vi "DAQmx.Stop.vi"(8 "error in (no error)":errorcluster, 11 "DAQmx in":refnum<class "DAQmx.lvclass">) -> (0 "error out":errorcluster, 3 "DAQmx out":refnum<class "DAQmx.lvclass">)   [LabVIEW 2019, in "DAQmx.lvclass"]
uses:
  DAQmx.lvclass
  DAQmx.lvclass/DAQmx.ctl
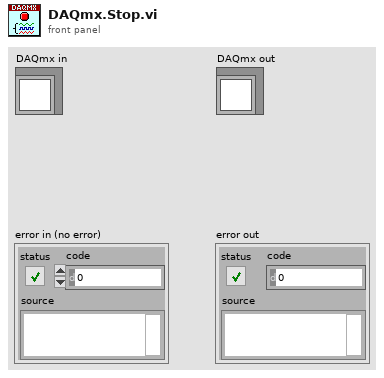
[diagram p1: front panel]
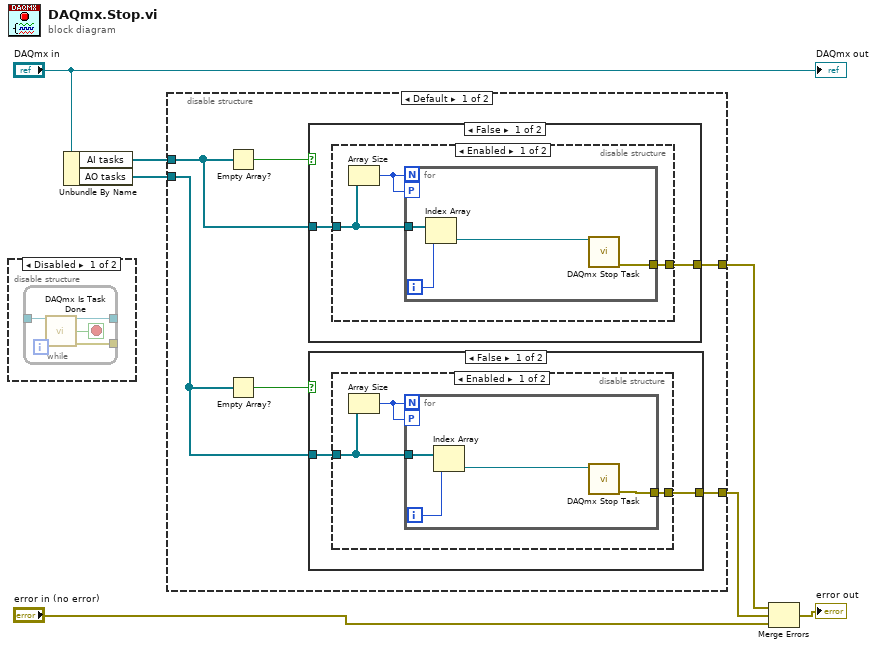
[diagram p0: block diagram]
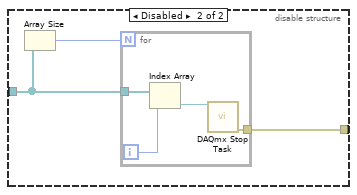
[diagram p3: hidden frame]
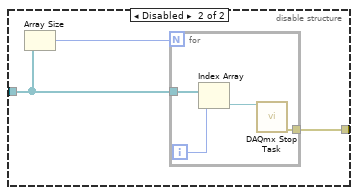
[diagram p5: hidden frame]
diagram:
  n1 = disable-structure shown="Disabled" {
    frame Disabled {
      n2 = while {
        tunnel: [w9] -> _
        tunnel: _ -> [w11]
        tunnel: [w10] -> _
        stop <- w8 stop-if-true
        n3 = call <vilib>:"DAQmx Is Task Done.vi"("task/channels in"=w11) -> ("task out"=w10:refnum<k21>, "task done?"=w8:bool, "error out"=w9:errorcluster)  [unwired: 12 in]
      }
    }
    frame Enabled {
    }
  }
  n4 = Unbundle By Name("DAQmx in") -> ("AI tasks"=w6:refnum<k21>[], "AO tasks"=w7:refnum<k21>[])
  n5 = disable-structure shown="Default" {
    disable-tunnel: [w17 _] -> w3
    disable-tunnel: w7 -> [w13 _]
    disable-tunnel: w6 -> [w15 _]
    disable-tunnel: [w12 _] -> w1
    frame condition #0 (active) {
      n6 = Empty Array?(array=w15) -> (empty?=w16:bool)
      n7 = Empty Array?(array=w13) -> (empty?=w14:bool)
      n8 = case shown="False" w16 {
        tunnel: w15 -> [w34 _]
        tunnel: [w35 _] -> w17
        frame False {
          n9 = disable-structure shown="Enabled" {
            disable-tunnel: [w38 w45] -> w35
            disable-tunnel: w34 -> [w37 w44]
            frame Enabled {
              n10 = Array Size(array=w37) -> (size(s)=w36:i32)
              n11 = for {
                N: w36 -> [_]
                tunnel: w37 -> [w41]
                tunnel: [w42] -> w38
                workers-P: w36 -> [_]
                i -> [w40]
                n12 = Index Array(array=w41, index=w40) -> (element=w39:refnum<k21>)
                n13 = call <vilib>:"DAQmx Stop Task.vi"("task/channels in"=w39) -> ("error out"=w42:errorcluster)  [unwired: 13 in, 1 out]
              }
            }
            frame Disabled {
              n14 = Array Size(array=w44) -> (size(s)=w43:i32)
              n15 = for {
                N: w43 -> [_]
                tunnel: w44 -> [w48]
                tunnel: [w49] -> w45
                i -> [w47]
                n16 = Index Array(array=w48, index=w47) -> (element=w46:refnum<k21>)
                n17 = call <vilib>:"DAQmx Stop Task.vi"("task/channels in"=w46) -> ("error out"=w49:errorcluster)  [unwired: 13 in, 1 out]
              }
            }
          }
        }
        frame True {
        }
      }
      n18 = case shown="False" w14 {
        tunnel: w13 -> [w18 _]
        tunnel: [w19 _] -> w12
        frame False {
          n19 = disable-structure shown="Enabled" {
            disable-tunnel: [w22 w29] -> w19
            disable-tunnel: w18 -> [w21 w28]
            frame Enabled {
              n20 = Array Size(array=w21) -> (size(s)=w20:i32)
              n21 = for {
                N: w20 -> [_]
                tunnel: w21 -> [w25]
                tunnel: [w26] -> w22
                workers-P: w20 -> [_]
                i -> [w24]
                n22 = Index Array(array=w25, index=w24) -> (element=w23:refnum<k21>)
                n23 = call <vilib>:"DAQmx Stop Task.vi"("task/channels in"=w23) -> ("error out"=w26:errorcluster)  [unwired: 13 in, 1 out]
              }
            }
            frame Disabled {
              n24 = Array Size(array=w28) -> (size(s)=w27:i32)
              n25 = for {
                N: w27 -> [_]
                tunnel: w28 -> [w32]
                tunnel: [w33] -> w29
                i -> [w31]
                n26 = Index Array(array=w32, index=w31) -> (element=w30:refnum<k21>)
                n27 = call <vilib>:"DAQmx Stop Task.vi"("task/channels in"=w30) -> ("error out"=w33:errorcluster)  [unwired: 13 in, 1 out]
              }
            }
          }
        }
        frame True {
        }
      }
    }
    frame condition #1 {
    }
  }
  n28 = Merge Errors(w3, w1, "error in (no error)") -> (→"error out":errorcluster)
  "DAQmx out" <- "DAQmx in"
